vi "DG Calculate Fit.vi"(8 "error in (no error)":errorcluster, 10 "DG measurement":T1={"Signal frequencies (Hz)"=[1000.0], "Signal amplitudes (V)"=[0.707], "Sampling frequencies (Hz)"=[10000000.0], "Record lengths (multiples of periods)"=[10000.0], "Calculate results"=FALSE, "Algorithm"="TWM-PJVSSubS", "TWM data directories"=[], "TWM data directories relative"=[], "PJVS frequencies (Hz)"=[1000.0], "PJVS reference voltages array of vector cluster"=[], "Requested PJVS steps"=[20], "Data folder"=path "", "Rs"=0, "Re"=0, "Settle down after PJVS change (s)"=1.0, "Switch position"=0.0, "PJVS amplitudes (Hz)"=[1000.0], "DG measurement info files"=[]} {"PJVS amplitudes (Hz)" format="%#_3p"; "PJVS reference voltages array of vector cluster"."PJVS reference voltages vector" format="%#_3p"; "PJVS frequencies (Hz)" format="%#_3p"; "Record lengths (multiples of periods)" format="%#_3p"; "Sampling frequencies (Hz)" format="%#_3p"; "Signal amplitudes (V)" format="%#_3p"; "Signal frequencies (Hz)" format="%#_3p"}, 11 "Common properties":T2={"Measurement status ref"=refnum, "TWM Status ref"=refnum, "Abort ref"=refnum, "Skip waiting ref"=refnum, "GNU Octave path"=path "C:/Program Files/GNU Octave/Octave-6.2.0/mingw64/bin", "TWM+QWTB path"=path "C:/Users/labina/Desktop/TWM-1.8.7.0-full/octprog", "lvlib path"=path "D:/martin/WAC/WACsw - github/control_software/Filter function meter/external libraries/GOLPI 0.7.3.1 source distribution LV 20.0 32 bit/lv_proc.dll", "TWM pipe"="\\\\.\\pipe\\TWM:server", "PJVS status ref"=refnum, "WAC path"=path ""}) -> (0 "error out":errorcluster)   [LabVIEW 2020]
doc: "Runs calculation of CE measurement using read_M_CE_from_spreadsheet.m and P_CE.m scripts."
uses:
  external libraries/GOLPI 0.7.3.1 source distribution LV 20.0 32 bit/GOLPI library.lvlib
  Utilities/Calculation related/Globals for GOLPI.vi
  Utilities/Type definitions/Common properties.ctl
  DG Measurement/DG measurement.ctl
panel:
  out "command\n(for debug)":string="addpath('info'); addpath('qwtb'); qwtb_exec_algorithm('%s', 0, 1); disp('FINISHEDCR')"
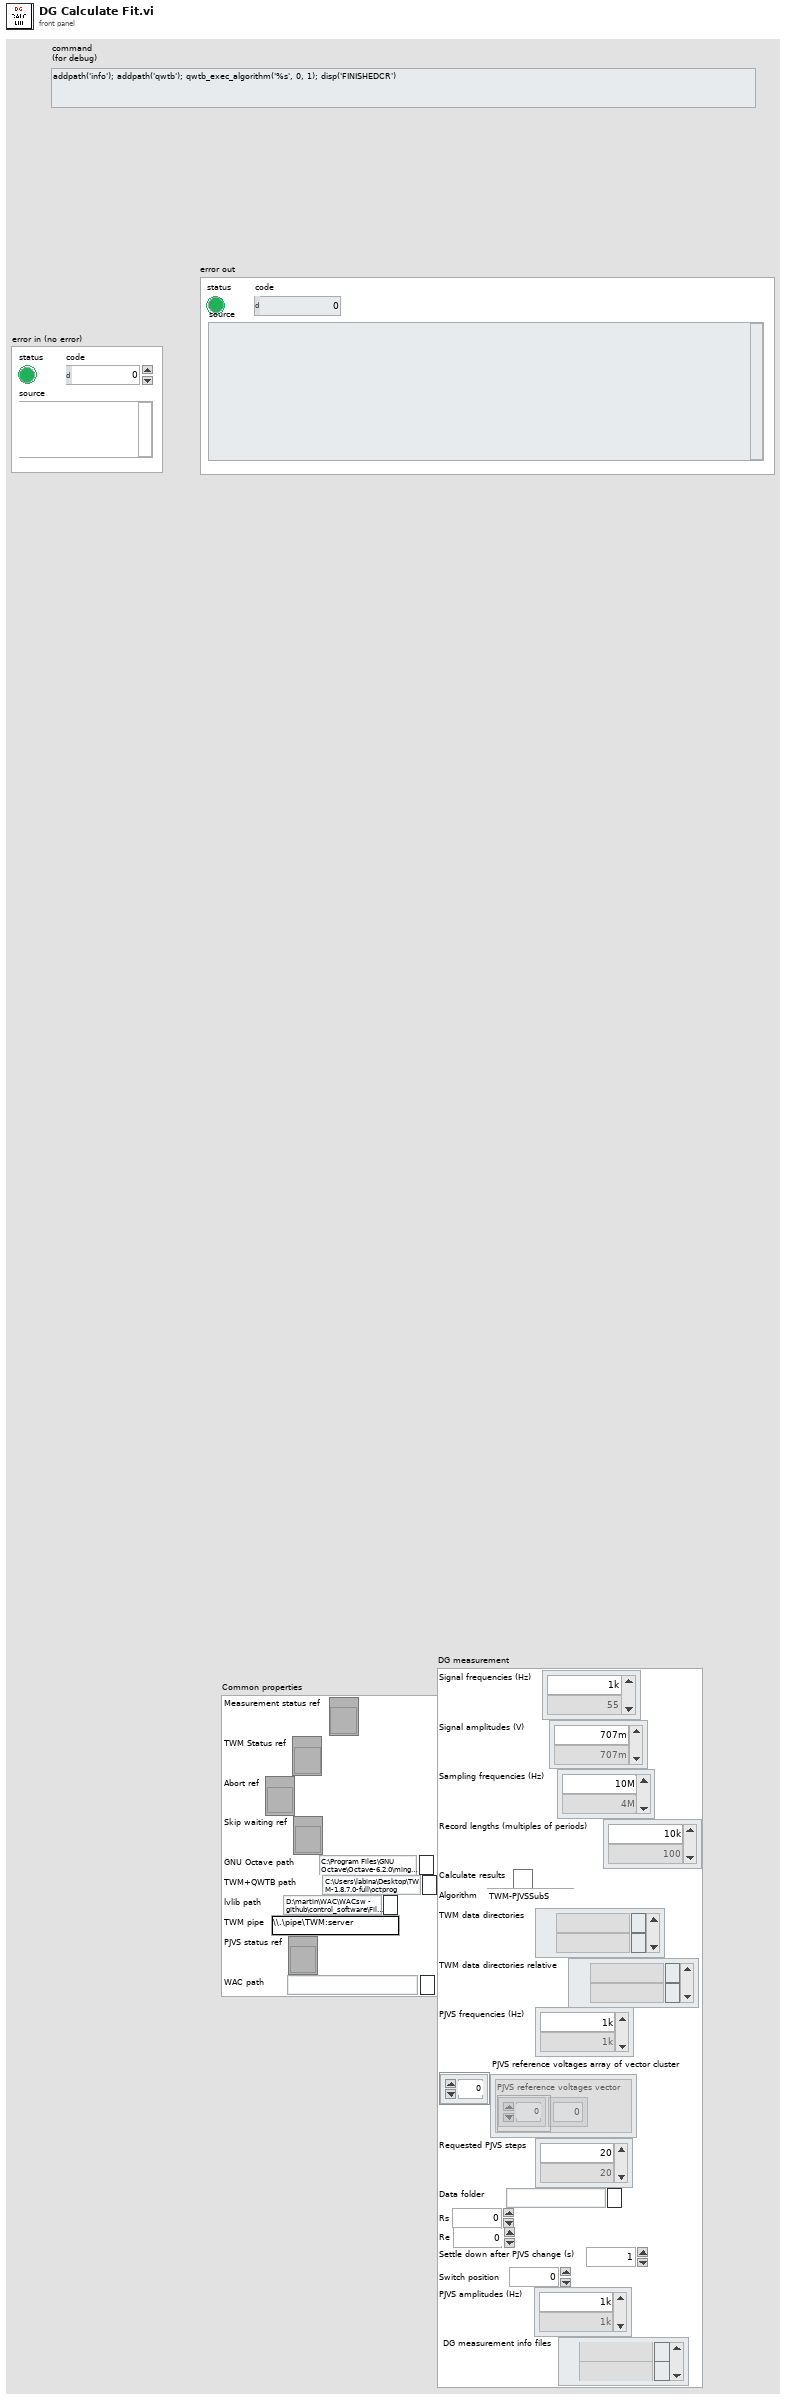
[diagram p1: front panel]
types:
  T1 = typedef "DG measurement.ctl" = cluster{"Signal frequencies (Hz)":dbl[], "Signal amplitudes (V)":dbl[], "Sampling frequencies (Hz)":dbl[], "Record lengths (multiples of periods)":dbl[], "Calculate results":bool, "Algorithm":string, "TWM data directories":path[], "TWM data directories relative":path[], "PJVS frequencies (Hz)":dbl[], "PJVS reference voltages array of vector cluster":cluster{"PJVS reference voltages vector":dbl[]}[], "Requested PJVS steps":u32[], "Data folder":path, "Rs":i32, "Re":i32, "Settle down after PJVS change (s)":dbl, "Switch position":dbl, "PJVS amplitudes (Hz)":dbl[], "DG measurement info files":path[]}
  T2 = typedef "Common properties.ctl" = cluster{"Measurement status ref":refnum<vi>, "TWM Status ref":refnum<vi>, "Abort ref":refnum<vi>, "Skip waiting ref":refnum<vi>, "GNU Octave path":path, "TWM+QWTB path":path, "lvlib path":path, "TWM pipe":string, "PJVS status ref":refnum<vi>, "WAC path":path}
  T3 = typedef "GOLPI library.lvlib/GOLPI reference Type Def.ctl" = cluster{"pipe handle":T4, "fast read timeout [ms]":u32, "fast read settle time [ms]":u32, "fast read to multiple [ms]":u32, "max elements per input line":u32, "slow read timeout [ms]":u32, "stdin double format specifier":string, "max elements per stdout output column":u32, "console mode bitstream":bool, "bitstream first read timeout [ms]":u32, "bitstream read timeout [ms]":u32, "struct transfer possible":bool, "matlab mode":bool}
  T4 = typedef "LV Process library.lvlib/Pipe Handle.ctl" = cluster{"lv_proc.dll file path":path, "process instance handle":u32[], "debug mode":bool, "debug data":cluster{"time":timestamp, "stdin":bool, "data":string}[]}
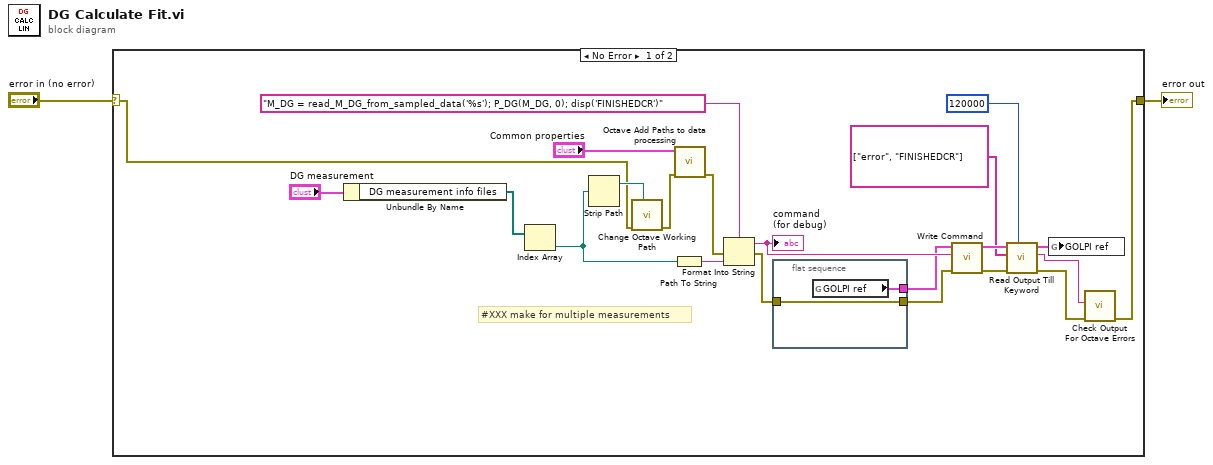
[diagram p0: block diagram]
diagram:
  n1 = case shown="No Error" "error in (no error)" {
    selector: "error in (no error)" -> [w16 w27]
    tunnel: [w7 w27] -> w2
    frame No Error {
      # "#XXX make for multiple measurements"
      n2 = Unbundle By Name("DG measurement") -> ("DG measurement info files"=w4:path[])
      n3 = Index Array(array=w4) -> (element=w3:path)  [unwired: 1 in]
      n4 = Strip Path(path=w3) -> (stripped path=w17:path)  [unwired: 1 out]
      n5 = call "Change Octave Working Path.vi"("Measurement path in"=w17, "error in (no error)"=w16) -> ("error out"=w11:errorcluster)  [unwired: 9 in]
      n6 = Path To String(path=w3) -> (string=w23:string)
      n7 = call "Octave Add Paths to data processing.vi"("error in (no error)"=w11, "Common properties"="Common properties") -> ("error out"=w10:errorcluster)  [unwired: 9 in]
      n8 = Format Into String(format string="M_DG = read_M_DG_from_sampled_data('%s'); P_DG(M_DG, 0); disp('FINISHEDCR')", error in=w10, w23) -> (resulting string=w18:string, error out=w15:errorcluster)  [unwired: 1 in]
      "command\n(for debug)" <- w18
      n9 = flat-sequence {
        tunnel: [w26] -> w14
        tunnel: w15 -> [w26]
        tunnel: [w25] -> w13
        frame #0 {
          n10 = global read "Globals for GOLPI.vi" "GOLPI ref"() -> (w25:T3)
        }
      }
      n11 = call "Write Command.vi"("error in"=w14, "command"=w18, "GOLPI ref. in"=w13) -> ("error out"=w22:errorcluster, "GOLPI ref. out"=w21:T3)  [unwired: 7 in]
      n12 = call "Read Output Till Keyword.vi"("timeout [ms]"=u32 120000, "error in"=w22, "keywords"=string[] ["error", "FINISHEDCR"], "GOLPI ref. in"=w21) -> ("error out"=w8:errorcluster, "read buffer"=w6:string, "GOLPI ref. out"=w12:T3)  [unwired: 4 in, 1 out]
      n13 = global write "Globals for GOLPI.vi" "GOLPI ref"(w12) -> ()
      n14 = call "Check Output For Octave Errors.vi"("error in"=w8, "read buffer"=w6) -> ("error out"=w7:errorcluster)  [unwired: 9 in]
    }
    frame Error {
    }
  }
  "error out" <- w2
